vi "Read PumpState.vi"(11 "Pump_1AI_1DO_2DI in":refnum<class "Engine_1DI_2DO.lvclass">) -> (2 "PumpState":T1)   [LabVIEW 2019, in "Engine_1DI_2DO.lvclass"]
uses:
  Engine_1DI_2DO.lvclass
  TypeDef/StatePump.ctl
  Engine_1DI_2DO.lvclass/Engine_1DI_2DO.ctl
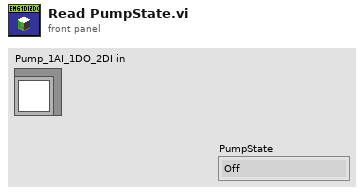
[diagram p1: front panel]
types:
  T1 = typedef "StatePump.ctl" = enum16{"Off", "TupningOn", "On", "TurningOff"}
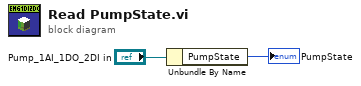
[diagram p0: block diagram]
diagram:
  n1 = Unbundle By Name("Pump_1AI_1DO_2DI in") -> ("PumpState"=→"PumpState":T1)
